vi "Get Digital Demod Trace Name.vi"(8 "error in (no error)":errorcluster {"code" format="%.0x"}, 9 "NameBufferSize":i32=256, 10 "Index":i32 format="%.0g", 11 "instrument handle":refnum<k15>) -> (0 "error out":errorcluster {"code" format="%.0x"}, 2 "Name":string, 3 "instrument handle out":refnum<k15>)   [LabVIEW 2021, in "Keysight XSAnVMA.lvlib"]
doc: "Returns the digitaldemodtrace name that corresponds to the one-based index that the user specifies."
uses:
  <instrlib>/Keysight XSAnVMA/Keysight XSAnVMA.lvlib
  KtXSAnVMA_64.dll
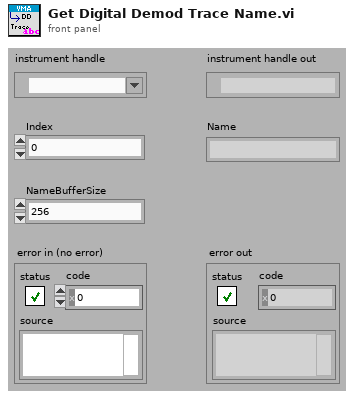
[diagram p1: front panel]
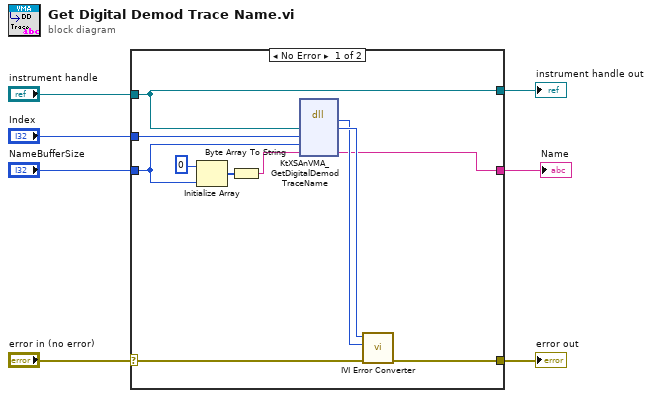
[diagram p0: block diagram]
diagram:
  n1 = case shown="No Error" "error in (no error)" {
    selector: "error in (no error)" -> [w16 w20]
    tunnel: [w15 w20] -> w7
    tunnel: "instrument handle" -> [w8 w19]
    tunnel: "Index" -> [w14 _]
    tunnel: "NameBufferSize" -> [w9 _]
    tunnel: [w10 _] -> w2
    tunnel: [w8 w19] -> w1
    frame No Error {
      n2 = Initialize Array(u8 0 ("element"), w9) -> (w12:u8[])
      n3 = Byte Array To String(unsigned byte array=w12) -> (string=w13:string)
      n4 = dll-call lib="KtXSAnVMA**.dll" fn="KtXSAnVMA_GetDigitalDemodTraceName"("Vi"=w8, "Index"=w14, "NameBufferSize"=w9, "Name"=w13) -> (w17:i32, "Vi"=w18:u32, "Name"=w10:string)  [unwired: 5 in, 2 out]
      n5 = call <instrlib>:"IVI Error Converter.vi"("error in (no error)"=w16, "IVI error code (0)"=w17, "instrument handle"=w18) -> ("error out"=w15:errorcluster)  [unwired: 7 in, 1 out]
    }
    frame Error {
    }
  }
  "error out" <- w7
  "instrument handle out" <- w1
  "Name" <- w2
